vi "ModifyClassAttribute.vi"(5 "error in (no error)":errorcluster) -> (16 "created new":bool, 19 "error out":errorcluster)   [LabVIEW 2017, in "G#StaticClass.lvclass"]
uses:
  G#StaticClass.lvclass
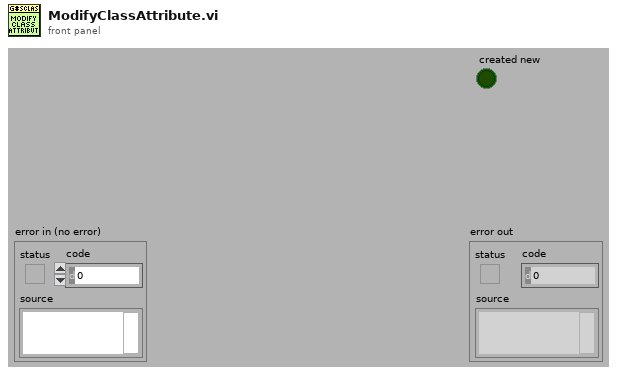
[diagram p1: front panel]
types:
  T1 = typedef "G#StaticClass.lvclass/ClassAttributesRef.ctl" = refnum<data-value>
  T2 = typedef "G#StaticClass.lvclass/ClassAttributes.ctl" = cluster{"Static":i32}
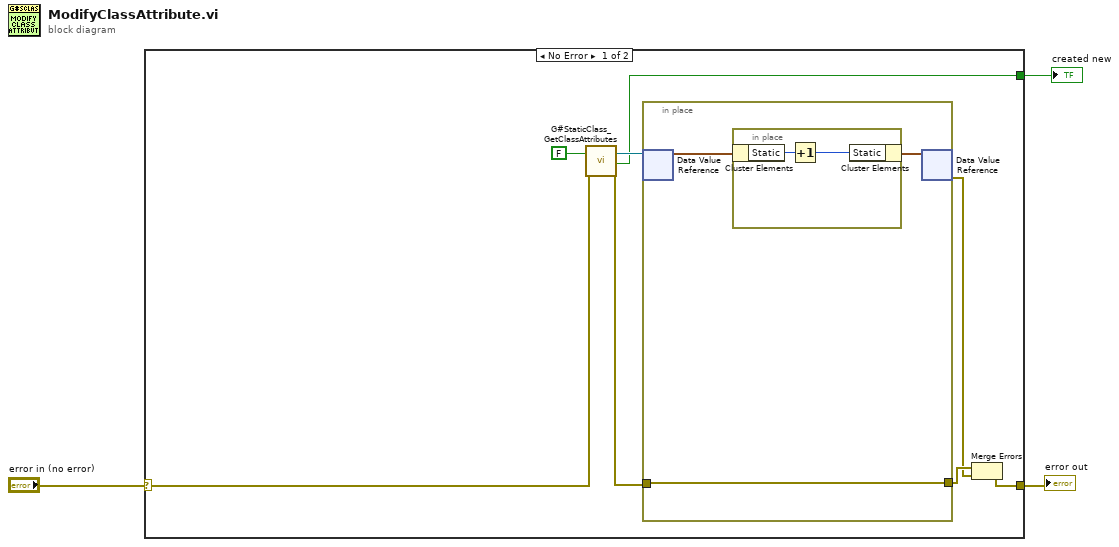
[diagram p0: block diagram]
diagram:
  n1 = case shown="No Error" "error in (no error)" {
    selector: "error in (no error)" -> [w11 w17]
    tunnel: [w8 w17] -> w2
    tunnel: [w4 _] -> w1
    frame No Error {
      n2 = call "G#StaticClass_GetClassAttributes.vi"("return data? (T)"=FALSE ("return data"), "error in (no error)"=w11) -> ("class attributes ref"=w9:T1, "created new"=w4:bool, "error out"=w10:errorcluster)  [unwired: 14 in, 1 out]
      n3 = in-place {
        in-place-border: w10 -> [w12]
        in-place-border: [w12] -> w6
        n4 = in-place-dvr #1(w9) -> (w13:T2)  [unwired: 1 out]
        n5 = in-place {
          n6 = in-place-cluster #2(w13) -> ("Static"=w16:i32)
          n7 = Increment(x=w16) -> (x+1=w15:i32)
          n8 = in-place-cluster #2("Static"=w15) -> (w14:T2)
        }
        n9 = in-place-dvr #1(w14) -> (w5:errorcluster)  [unwired: 1 out]
      }
      n10 = Merge Errors(w6, w5) -> (w8:errorcluster)
    }
    frame Error {
    }
  }
  "error out" <- w2
  "created new" <- w1
